vi "fpga_main.vi"() -> ()   [LabVIEW 2024]
uses:
  FPGA_Operation_Control.ctl
  PWM Counter Selector.ctl
  <vilib>/rvi/Emulation/niFpgaGetClockAttributes.vi
  <vilib>/rvi/Emulation/niFpgaSctlEmulationGetInTimedLoop.vi
  <vilib>/rvi/Emulation/niFpgaEmulationReportErrorSimple.vi
  <vilib>/rvi/Emulation/niFpgaEmulationIsFPGAContextNoSignature.vi
  <vilib>/rvi/DataTransferAndStorage/Container/Common/niFpgaContainerGetUniqueNameForEmu.vi
  <vilib>/rvi/Memory/Memory_Emulation/niFpgaMemoryEmulationCacheClearOnFirstRun.vi
  <vilib>/rvi/Memory/Memory_Emulation/nirvimemoryEmulationManagerCache_MakeExclusive.vi
  <vilib>/rvi/Memory/Memory_Emulation/niFpgaMemoryEmulationValidateCache.vi
  <vilib>/rvi/Memory/Memory_Emulation/nirvimemoryEmulationManagerCache_InsertValue.vi
  <vilib>/Utility/error.llb/Clear Errors.vi
  <vilib>/rvi/Memory/Memory_Emulation/nirvimemoryEmulationManagerCache_ReleaseExclusive.vi
  <vilib>/rvi/Memory/Memory_Emulation/nirvimemoryEmulationManagerCache_GetValue.vi
  <vilib>/rvi/Memory/Memory_Emulation/nirvimemoryEmulationManagerCache_SetValue.vi
  <vilib>/rvi/Emulation/niFpgaProcessEmulError.vi
  <vilib>/rvi/Emulation/niFpgaCriticalErrorInLSC.vi
  <vilib>/rvi/DataTransferAndStorage/Container/XNode/niFpgaContainer.xnode
  <vilib>/rvi/DataTransferAndStorage/Register/Emulation/niFpgaRegisterEmulation.vi
panel:
  in  "R/W":bool
  in  "INPUT":u8
  out "OUTPUT":i16
  in  "OPERATION":T1
  in  "ENABLE":bool
  in  "PIN":u8
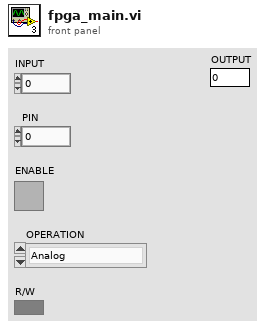
[diagram p1: front panel]
types:
  T1 = typedef "FPGA_Operation_Control.ctl" = enum16{"Analog", "Digital", "PWM"}
  T2 = typedef "PWM Counter Selector.ctl" = enum16{"Not in use", "PWM 1", "PWM 2", "PWM 3", "PWM 4", "PWM 5", "PWM 6", "PWM 7", "PWM 8"}
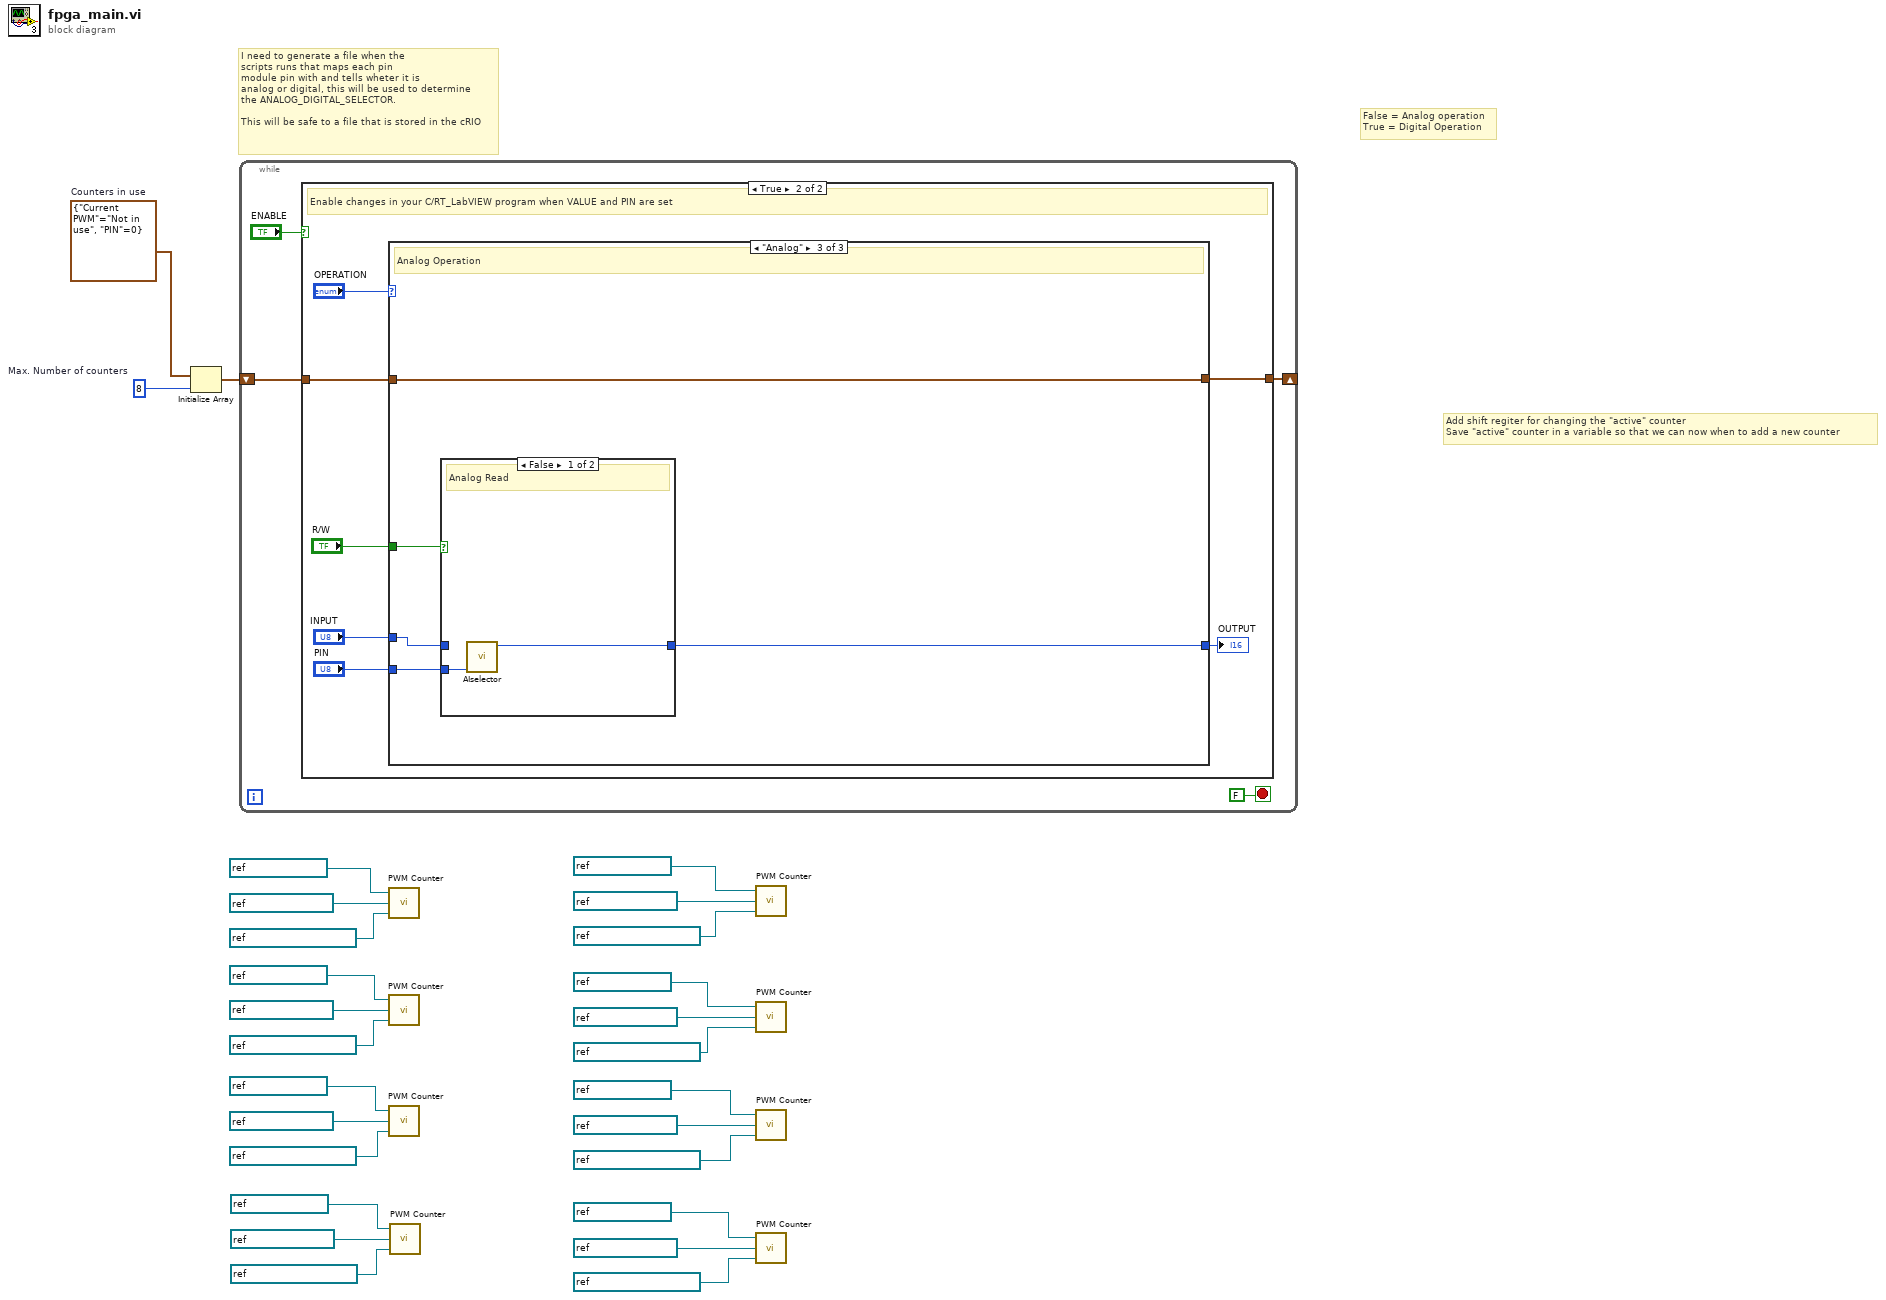
[diagram p0: block diagram]
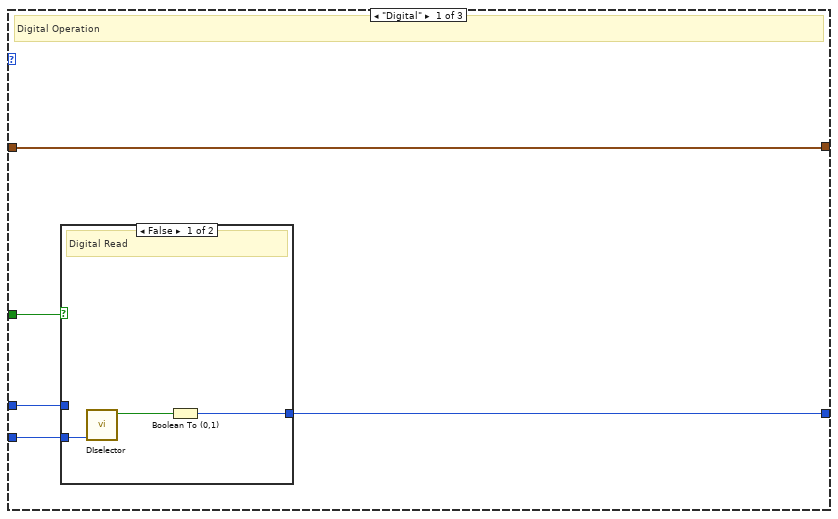
[diagram p3: hidden frame]
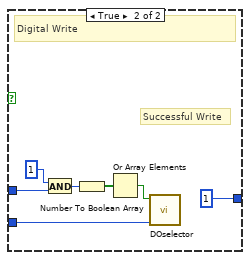
[diagram p4: hidden frame]
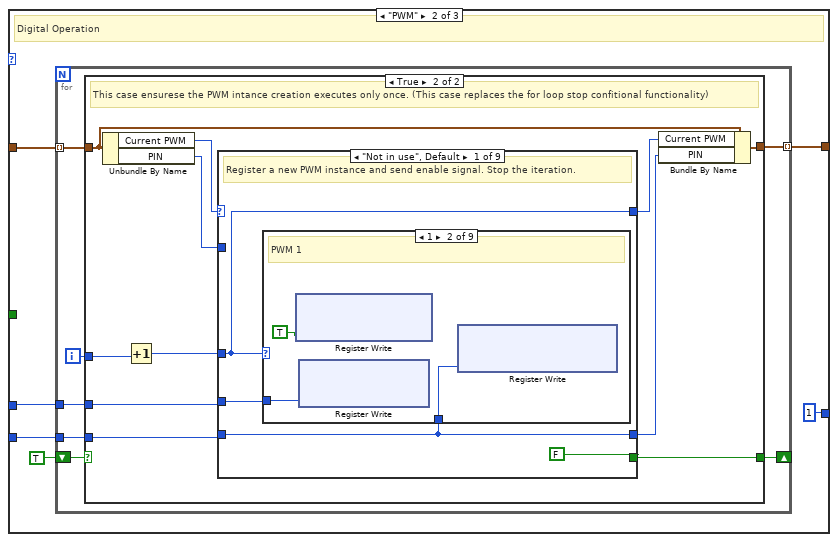
[diagram p5: hidden frame]
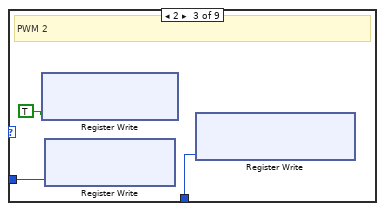
[diagram p8: hidden frame]
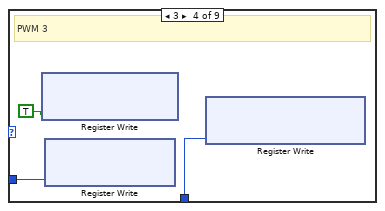
[diagram p9: hidden frame]
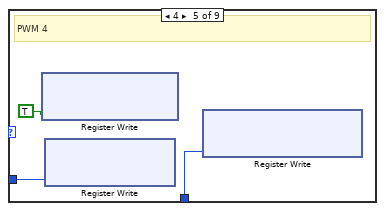
[diagram p10: hidden frame]
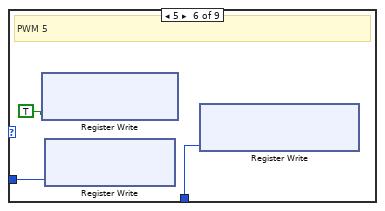
[diagram p11: hidden frame]
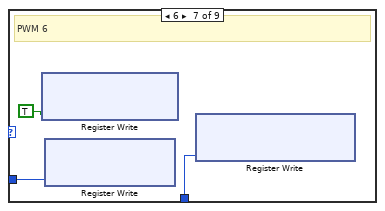
[diagram p12: hidden frame]
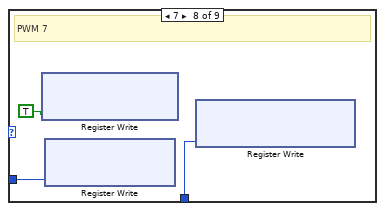
[diagram p13: hidden frame]
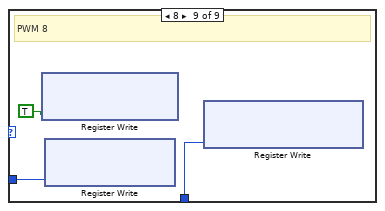
[diagram p14: hidden frame]
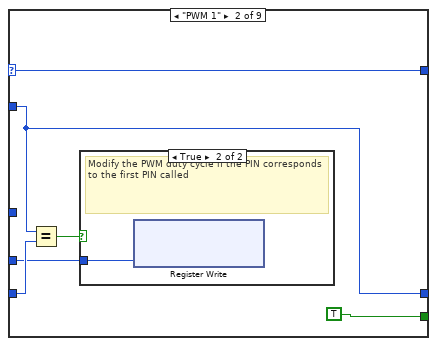
[diagram p15: hidden frame]
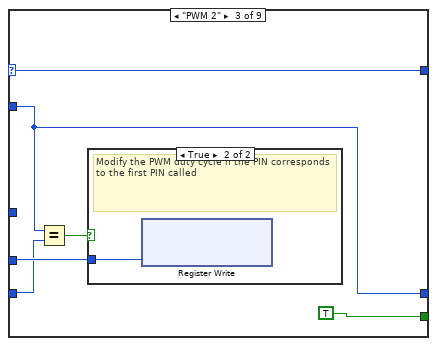
[diagram p17: hidden frame]
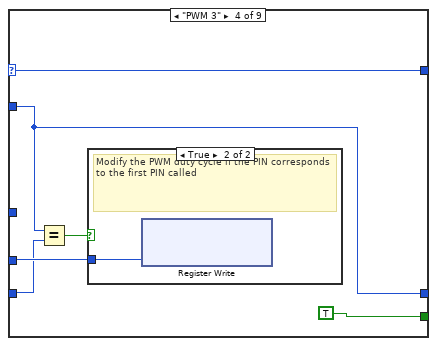
[diagram p19: hidden frame]
diagram:
  w26 = cluster{"Current PWM":T2, "PIN":u8} {"Current PWM"=enum."Not in use", "PIN"=0}  # Counters in use
  w27 = 8  # Max. Number of counters
  # "Add shift regiter for changing the \"active\" counter\nSave \"active\" counter in a variable so that we can now when to add a new counter"
  # "False = Analog operation\nTrue = Digital Operation"
  # "I need to generate a file when the \nscripts runs that maps each pin\nmodule pin with and tells wheter it is\nanalog or digital, this will be used to determine\nthe ANALOG_DIGITAL_SELECTOR.\n\nThis will be safe to a file that is stored in the cRIO"
  n1 = Initialize Array(w26, w27) -> (w25:cluster{"Current PWM":T2, "PIN":u8}[])
  n2 = while {
    shift-right: [w29] -> _
    shift-left: w25 -> [w28]
    stop <- FALSE stop-if-true
    n3 = case shown="True" "ENABLE" {
      tunnel: w28 -> [w32 w37]
      tunnel: [w32 w34] -> w29
      frame False {
      }
      frame True {
        # "Enable changes in your C/RT_LabVIEW program when VALUE and PIN are set"
        n4 = case shown="\"Analog\"" "OPERATION" {
          tunnel: "PIN" -> [w44 w59 w169]
          tunnel: "INPUT" -> [w43 w58 w168]
          tunnel: w37 -> [w42 w60 w167]
          tunnel: [w42 w56 w167] -> w34
          tunnel: "R/W" -> [w41 _ w165]
          tunnel: [w40 i16 1 ("value") w166] -> w35
          frame "Digital" {
            # "Digital Operation"
            n5 = case shown="False" w41 {
              tunnel: w44 -> [w47 w54]
              tunnel: w43 -> [_ w53]
              tunnel: [w45 i16 1] -> w40
              frame False {
                # "Digital Read"
                n6 = call "DIselector.vi"("I/O element"=w47) -> ("value"=w46:bool)  [unwired: 10 in]
                n7 = Boolean To (0,1)(Boolean=w46) -> (0, 1=w45:i16)
              }
              frame True {
                # "Successful Write"
                # "Digital Write"
                n8 = And(x=u8 1, y=w53) -> (x .and. y?=w51:u8)
                n9 = Number To Boolean Array(number=w51) -> (Boolean array=w49:bool[])
                n10 = Or Array Elements(Boolean array=w49) -> (logical OR=w50:bool)
                n11 = call "DOselector.vi"("I/O element"=w54, "value"=w50) -> ()  [unwired: 10 in]
              }
            }
          }
          frame "PWM" {
            # "Digital Operation"
            n12 = for {
              tunnel: w60 -> [w67] mode=indexing
              tunnel: w59 -> [w66]
              tunnel: w58 -> [w64]
              shift-right: [w63] -> _
              shift-left: TRUE -> [w62]
              tunnel: [w61] -> w56 mode=indexing
              i -> [w65]
              n13 = case shown="True" w62 {
                selector: w62 -> [w68 _]
                tunnel: w67 -> [w69 w80]
                tunnel: w66 -> [_ w74]
                tunnel: w65 -> [_ w76]
                tunnel: w64 -> [_ w75]
                tunnel: [w68 w70] -> w63
                tunnel: [w69 w79] -> w61
                frame False {
                }
                frame True {
                  # "This case ensurese the PWM intance creation executes only once. (This case replaces the for loop stop confitional functionality)"
                  n14 = Unbundle By Name(w80) -> ("Current PWM"=w73:T2, "PIN"=w72:u8)
                  n15 = Increment(x=w76) -> (x+1=w78:i32)
                  n16 = case shown="\"Not in use\", Default" w73 {
                    selector: w73 -> [_ w110 w118 w125 w132 w139 w146 w153 w160]
                    tunnel: w74 -> [w82 w114 w119 w126 w133 w140 w147 w154 w161]
                    tunnel: [w82 w109 w116 w123 w130 w137 w144 w151 w158] -> w77
                    tunnel: w78 -> [w84 _ _ _ _ _ _ _ _]
                    tunnel: [w84 w110 w118 w125 w132 w139 w146 w153 w160] -> w71
                    tunnel: w75 -> [w83 w112 w120 w127 w134 w141 w148 w155 w162]
                    tunnel: [FALSE TRUE TRUE TRUE TRUE TRUE TRUE TRUE TRUE] -> w70
                    tunnel: w72 -> [_ w109 w116 w123 w130 w137 w144 w151 w158]
                    frame "Not in use", Default {
                      # "Register a new PWM instance and send enable signal. Stop the iteration."
                      n17 = case shown="1" w84 {
                        tunnel: w83 -> [_ w87 w90 w93 w96 w99 w102 w105 w108]
                        tunnel: w82 -> [_ w85 w88 w91 w94 w97 w100 w103 w106]
                        frame 0, Default {
                          # "Should never execute"
                        }
                        frame 1 {
                          # "PWM 1"
                          n18 = xnode ("Register Write")("Data"=TRUE) -> ()  [unwired: 1 in, 1 out]
                          n19 = xnode ("Register Write")("Data"=w87) -> ()  [unwired: 1 in, 1 out]
                          n20 = xnode ("Register Write")("Data"=w85) -> ()  [unwired: 1 in, 1 out]
                        }
                        frame 2 {
                          # "PWM 2"
                          n21 = xnode ("Register Write")("Data"=TRUE) -> ()  [unwired: 1 in, 1 out]
                          n22 = xnode ("Register Write")("Data"=w90) -> ()  [unwired: 1 in, 1 out]
                          n23 = xnode ("Register Write")("Data"=w88) -> ()  [unwired: 1 in, 1 out]
                        }
                        frame 3 {
                          # "PWM 3"
                          n24 = xnode ("Register Write")("Data"=TRUE) -> ()  [unwired: 1 in, 1 out]
                          n25 = xnode ("Register Write")("Data"=w93) -> ()  [unwired: 1 in, 1 out]
                          n26 = xnode ("Register Write")("Data"=w91) -> ()  [unwired: 1 in, 1 out]
                        }
                        frame 4 {
                          # "PWM 4"
                          n27 = xnode ("Register Write")("Data"=TRUE) -> ()  [unwired: 1 in, 1 out]
                          n28 = xnode ("Register Write")("Data"=w96) -> ()  [unwired: 1 in, 1 out]
                          n29 = xnode ("Register Write")("Data"=w94) -> ()  [unwired: 1 in, 1 out]
                        }
                        frame 5 {
                          # "PWM 5"
                          n30 = xnode ("Register Write")("Data"=TRUE) -> ()  [unwired: 1 in, 1 out]
                          n31 = xnode ("Register Write")("Data"=w99) -> ()  [unwired: 1 in, 1 out]
                          n32 = xnode ("Register Write")("Data"=w97) -> ()  [unwired: 1 in, 1 out]
                        }
                        frame 6 {
                          # "PWM 6"
                          n33 = xnode ("Register Write")("Data"=TRUE) -> ()  [unwired: 1 in, 1 out]
                          n34 = xnode ("Register Write")("Data"=w102) -> ()  [unwired: 1 in, 1 out]
                          n35 = xnode ("Register Write")("Data"=w100) -> ()  [unwired: 1 in, 1 out]
                        }
                        frame 7 {
                          # "PWM 7"
                          n36 = xnode ("Register Write")("Data"=TRUE) -> ()  [unwired: 1 in, 1 out]
                          n37 = xnode ("Register Write")("Data"=w105) -> ()  [unwired: 1 in, 1 out]
                          n38 = xnode ("Register Write")("Data"=w103) -> ()  [unwired: 1 in, 1 out]
                        }
                        frame 8 {
                          # "PWM 8"
                          n39 = xnode ("Register Write")("Data"=TRUE) -> ()  [unwired: 1 in, 1 out]
                          n40 = xnode ("Register Write")("Data"=w108) -> ()  [unwired: 1 in, 1 out]
                          n41 = xnode ("Register Write")("Data"=w106) -> ()  [unwired: 1 in, 1 out]
                        }
                      }
                    }
                    frame "PWM 1" {
                      n42 = Equal?(x=w109, y=w114) -> (x = y?=w113:bool)
                      n43 = case shown="True" w113 {
                        tunnel: w112 -> [_ w115]
                        frame False {
                        }
                        frame True {
                          # "Modify the PWM duty cycle if the PIN corresponds to the first PIN called"
                          n44 = xnode ("Register Write")("Data"=w115) -> ()  [unwired: 1 in, 1 out]
                        }
                      }
                    }
                    frame "PWM 2" {
                      n45 = Equal?(x=w116, y=w119) -> (x = y?=w121:bool)
                      n46 = case shown="True" w121 {
                        tunnel: w120 -> [_ w122]
                        frame False {
                          # "PIN is not the same. Do nothing"
                        }
                        frame True {
                          # "Modify the PWM duty cycle if the PIN corresponds to the first PIN called"
                          n47 = xnode ("Register Write")("Data"=w122) -> ()  [unwired: 1 in, 1 out]
                        }
                      }
                    }
                    frame "PWM 3" {
                      n48 = Equal?(x=w123, y=w126) -> (x = y?=w128:bool)
                      n49 = case shown="True" w128 {
                        tunnel: w127 -> [_ w129]
                        frame False {
                          # "PIN is not the same. Do nothing"
                        }
                        frame True {
                          # "Modify the PWM duty cycle if the PIN corresponds to the first PIN called"
                          n50 = xnode ("Register Write")("Data"=w129) -> ()  [unwired: 1 in, 1 out]
                        }
                      }
                    }
                    frame "PWM 4" {
                      n51 = Equal?(x=w130, y=w133) -> (x = y?=w135:bool)
                      n52 = case shown="True" w135 {
                        tunnel: w134 -> [_ w136]
                        frame False {
                          # "PIN is not the same. Do nothing"
                        }
                        frame True {
                          # "Modify the PWM duty cycle if the PIN corresponds to the first PIN called"
                          n53 = xnode ("Register Write")("Data"=w136) -> ()  [unwired: 1 in, 1 out]
                        }
                      }
                    }
                    frame "PWM 5" {
                      n54 = Equal?(x=w137, y=w140) -> (x = y?=w142:bool)
                      n55 = case shown="True" w142 {
                        tunnel: w141 -> [_ w143]
                        frame False {
                          # "PIN is not the same. Do nothing"
                        }
                        frame True {
                          # "Modify the PWM duty cycle if the PIN corresponds to the first PIN called"
                          n56 = xnode ("Register Write")("Data"=w143) -> ()  [unwired: 1 in, 1 out]
                        }
                      }
                    }
                    frame "PWM 6" {
                      n57 = Equal?(x=w144, y=w147) -> (x = y?=w149:bool)
                      n58 = case shown="True" w149 {
                        tunnel: w148 -> [_ w150]
                        frame False {
                          # "PIN is not the same. Do nothing"
                        }
                        frame True {
                          # "Modify the PWM duty cycle if the PIN corresponds to the first PIN called"
                          n59 = xnode ("Register Write")("Data"=w150) -> ()  [unwired: 1 in, 1 out]
                        }
                      }
                    }
                    frame "PWM 7" {
                      n60 = Equal?(x=w151, y=w154) -> (x = y?=w156:bool)
                      n61 = case shown="True" w156 {
                        tunnel: w155 -> [_ w157]
                        frame False {
                          # "PIN is not the same. Do nothing"
                        }
                        frame True {
                          # "Modify the PWM duty cycle if the PIN corresponds to the first PIN called"
                          n62 = xnode ("Register Write")("Data"=w157) -> ()  [unwired: 1 in, 1 out]
                        }
                      }
                    }
                    frame "PWM 8" {
                      n63 = Equal?(x=w158, y=w161) -> (x = y?=w163:bool)
                      n64 = case shown="True" w163 {
                        tunnel: w162 -> [_ w164]
                        frame False {
                          # "PIN is not the same. Do nothing"
                        }
                        frame True {
                          # "Modify the PWM duty cycle if the PIN corresponds to the first PIN called"
                          n65 = xnode ("Register Write")("Data"=w164) -> ()  [unwired: 1 in, 1 out]
                        }
                      }
                    }
                  }
                  n66 = Bundle By Name(cluster=w80, "Current PWM"=w71, "PIN"=w77) -> (w79:cluster{"Current PWM":T2, "PIN":u8})
                }
              }
            }
          }
          frame "Analog" {
            # "Analog Operation"
            n67 = case shown="False" w165 {
              tunnel: w169 -> [w171 w174]
              tunnel: w168 -> [_ w173]
              tunnel: [w170 i16 1 ("value")] -> w166
              frame False {
                # "Analog Read"
                n68 = call "AIselector.vi"("I/O element"=w171) -> ("value"=w170:i16)  [unwired: 10 in]
              }
              frame True {
                # "Successful\nWrite"
                # "Analog Write"
                n69 = call "AOselector.vi"("I/O element"=w174, "value"=w173) -> ()  [unwired: 10 in]
              }
            }
          }
        }
        "OUTPUT" <- w35
      }
    }
  }
  n70 = call "PWM Counter.vi"("PWM Output Pin"=refnum<k21> "PWM Output Pin 1", "PWM Enable"=refnum<k21> "PWM Enable 1", "PWM Value"=refnum<k21> "PWM Value 1") -> ()
  n71 = call "PWM Counter.vi"("PWM Output Pin"=refnum<k21> "PWM Output Pin 2", "PWM Enable"=refnum<k21> "PWM Enable 2", "PWM Value"=refnum<k21> "PWM Value 2") -> ()
  n72 = call "PWM Counter.vi"("PWM Output Pin"=refnum<k21> "PWM Output Pin 3", "PWM Enable"=refnum<k21> "PWM Enable 3", "PWM Value"=refnum<k21> "PWM Value 3") -> ()
  n73 = call "PWM Counter.vi"("PWM Output Pin"=refnum<k21> "PWM Output Pin 4", "PWM Enable"=refnum<k21> "PWM Enable 4", "PWM Value"=refnum<k21> "PWM Value 4") -> ()
  n74 = call "PWM Counter.vi"("PWM Output Pin"=refnum<k21> "PWM Output Pin 5", "PWM Enable"=refnum<k21> "PWM Enable 5", "PWM Value"=refnum<k21> "PWM Value 5") -> ()
  n75 = call "PWM Counter.vi"("PWM Output Pin"=refnum<k21> "PWM Output Pin 6", "PWM Enable"=refnum<k21> "PWM Enable 6", "PWM Value"=refnum<k21> "PWM Value 6") -> ()
  n76 = call "PWM Counter.vi"("PWM Output Pin"=refnum<k21> "PWM Output Pin 7", "PWM Enable"=refnum<k21> "PWM Enable 7", "PWM Value"=refnum<k21> "PWM Value 7") -> ()
  n77 = call "PWM Counter.vi"("PWM Output Pin"=refnum<k21> "PWM Output Pin 8", "PWM Enable"=refnum<k21> "PWM Enable 8", "PWM Value"=refnum<k21> "PWM Value 8") -> ()
